vi "run grafana.vi"(11 "working directory":path=path "C:/temp/grafana-v12.0.1 (2)/grafana-v12.0.1/bin") -> ()   [LabVIEW 2019]
panel:
  out "error out":errorcluster
  out "return code":i32
  out "standard error":string
  out "standard output":string
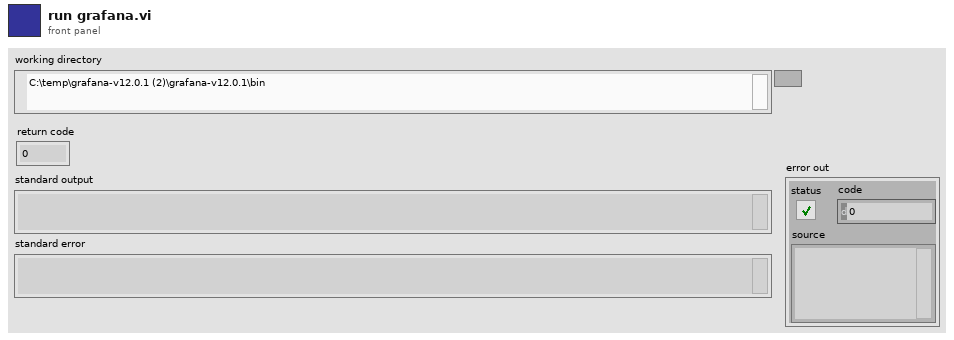
[diagram p1: front panel]
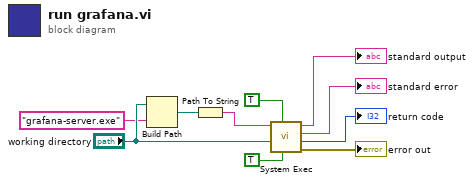
[diagram p0: block diagram]
diagram:
  n1 = Build Path(base path="working directory", name or relative path="grafana-server.exe" ("command line")) -> (appended path=w2:path)
  n2 = Path To String(path=w2) -> (string=w1:string)
  n3 = call <vilib>:"System Exec.vi"("run minimized? (F)"=TRUE, "wait until completion? (T)"=TRUE, "working directory"="working directory", "command line"=w1) -> ("error out"=→"error out":errorcluster, "return code"=→"return code":i32, "standard error"=→"standard error":string, "standard output"=→"standard output":string)  [unwired: 4 in]
